vi "Arrayindexing.vi.vi"() -> ()   [LabVIEW 2017]
panel:
  in  "cancel":bool
  out "Array":string[](array[string])
  in  "OK Button":bool
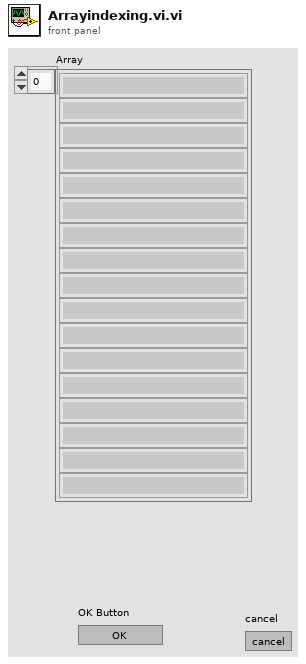
[diagram p1: front panel]
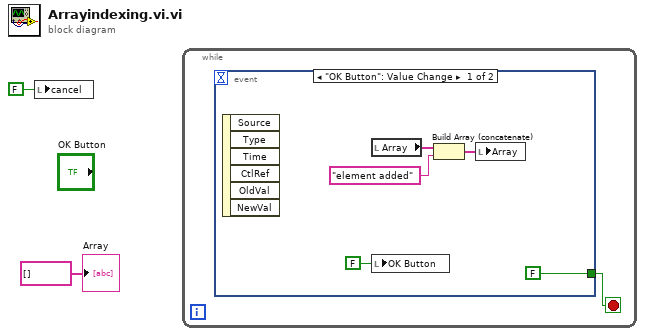
[diagram p0: block diagram]
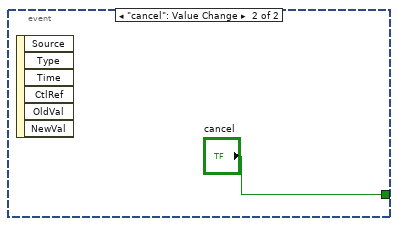
[diagram p2: hidden frame]
diagram:
  n1 = local write "cancel"(FALSE ("cancel")) -> ()
  n2 = while {
    stop <- w3 stop-if-true
    n3 = event shown="[0] \"OK Button\": Value Change" {
      selector: _ -> [_ _]
      dyn-events: _ -> [_ _]
      timeout: _ -> [_ _]
      tunnel: [FALSE ("cancel") "cancel"] -> w3
      event "OK Button": Value Change {
        n4 = event-data() -> ()  [unwired: 1 in, 6 out]
        n5 = local read "Array"() -> (w6:string[])
        n6 = local write "OK Button"(FALSE ("OK Button")) -> ()
        n7 = Build Array (concatenate)(w6, "element added" ("new element/subarray")) -> (w5:string[])
        n8 = local write "Array"(w5) -> ()
      }
      event "cancel": Value Change {
        n9 = event-data() -> ()  [unwired: 1 in, 6 out]
      }
    }
  }
  "Array" <- string[] [] ("Array")
